vi "SDG60ConfBurst2.vi"(0 "VISA resource name":refnum<visa-resource-name>="USB0::0xF4EC::0x1101::SDG6XEBC5R0119::INSTR", 1 "Trg/Gate Polarity 0: Rise/Pos":u16(ring) items=["Positive", "Negative"], 2 "Triggered/Gated: (0:Triggered)":i32(ring) items=["Triggered", "Gated"], 3 "TRG/Gate Source (0: Internal)":i32(ring) items=["Internal", "External", "Manual"], 5 "Enable Burst (T: Enable)":bool=TRUE, 7 "Channel (1:Channel 1)":i32(ring)=1 items=["Channel 1"=1, "Channel 2"=2], 9 "Start Phase (0.0 degrees)":dbl min=0.0 max=360.0 format="%#.15g", 10 "Burst Period (s)":dbl=1.352e-06, 11 "error in (no error)":errorcluster, 12 "Burst Delay (1.352 us)":dbl=1.352e-06, 13 "Burst Cycle (0: N-Cycle)":u16(ring) items=["N-Cycle", "Infinite"], 14 "Number of Cycles":i32=1) -> (4 "VISA resource name out":refnum<visa-resource-name>, 15 "error out":errorcluster)   [LabVIEW 2018]
panel:
  out "String":string
  # "Note: Ext TRG input is the same as output. TRG/Gate ext input has \nint pull up"
  # "Trigger values can't be changed\nTrigger High: 2-5.5V\nTrigger Low: -0.5-0.8V"
  # "Only positive works as it should\nSetting negative, still responds to rising edge and gives twice\nthe number of burst cycles with a delay. Don't use negative"
  # "Manual not possible in Gate, so\nauto sets to EXT"
  # "Range 1us-110ks. Min depends on freq\nValid and effective only for internal trig setting.\nAffects the period in external trg mode"
  # "Res: 0.1degrees\nRange: -280..+280 deg"
  # "Range: 1.352us-100s\nLimited by frequency\n6 digits precision"
  # "Burst delay also works as a delay with Gate via front panel Delay from triggered mode will be kept in gated mode. To change delay in gated, first need \nto set to triggered with delay time, then switch to gated"
  # "Non-standard behaviour!!: triggers are received while playing out a burst and lead to output of further partial bursts!! Some of these burst appear after burst period setting."
  # "Range: 1-2^31"
  # "When in external finite burst mode there is also a burst counter.\nIf set to >1 will produce multiple bursts with burst period that is\na leftover from triggered mode settnig. Default is 1, not controllable\nwithout using VKeys. Period is also not directly controllable."
  # "When in inf burst mode and ext triggered, the burst will start\nimmediately upon setting up  if external input is HI.\nSwitching output on and off resets inf burst."
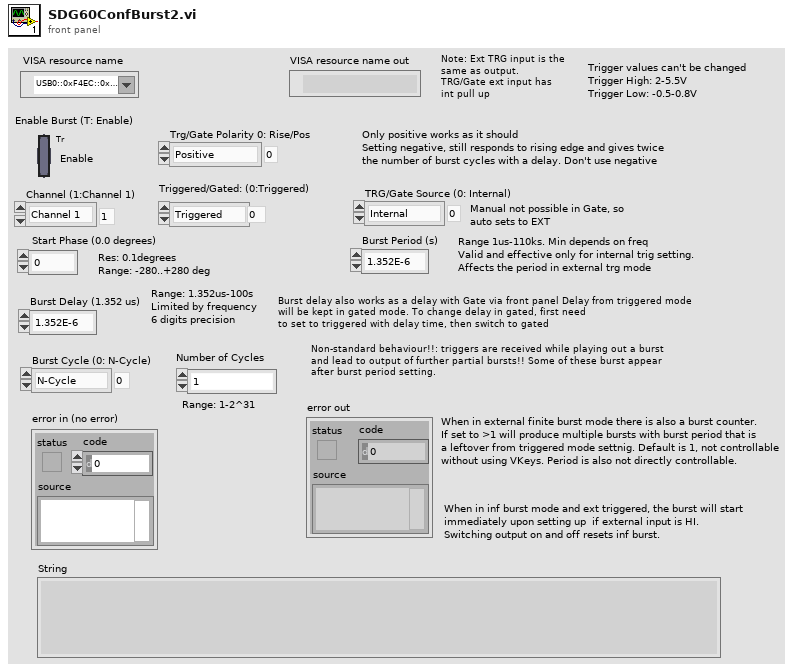
[diagram p1: front panel]
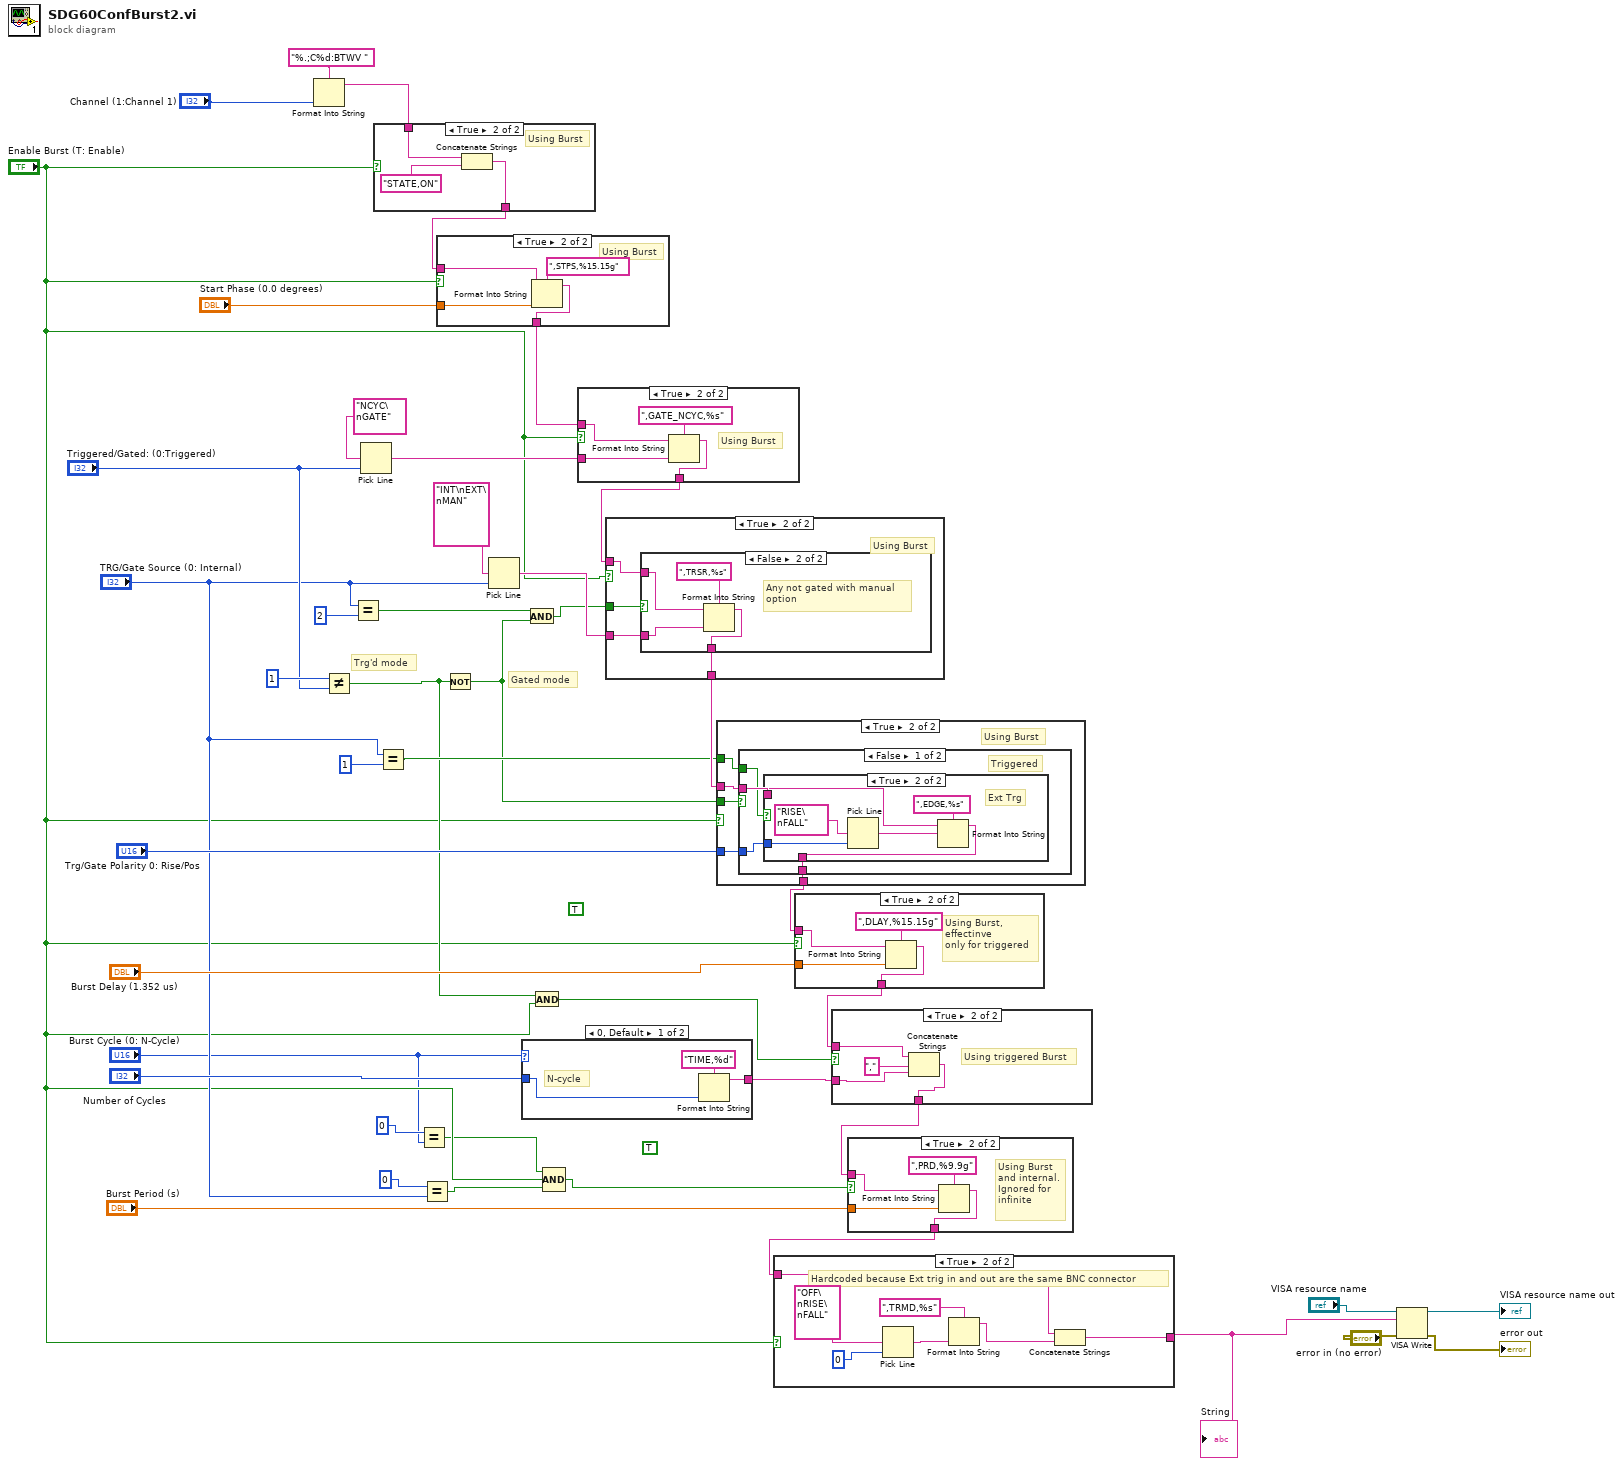
[diagram p0: block diagram]
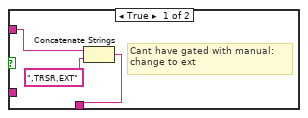
[diagram p4: hidden frame]
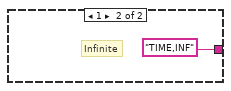
[diagram p6: hidden frame]
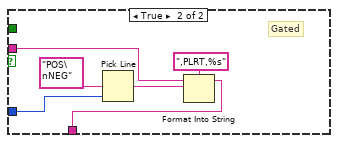
[diagram p10: hidden frame]
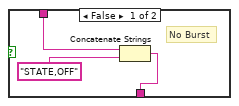
[diagram p14: hidden frame]
diagram:
  (unwired) TRUE
  (unwired) TRUE
  # "Trg'd mode"
  # "Gated mode"
  n1 = Format Into String(format string="%.;C%d:BTWV ", "Channel (1:Channel 1)") -> (resulting string=w42:string)  [unwired: 2 in, 1 out]
  n2 = Not Equal?(x=1, y="Triggered/Gated: (0:Triggered)") -> (x != y?=w7:bool)
  n3 = Equal?(x="TRG/Gate Source (0: Internal)", y=2) -> (x = y?=w15:bool)
  n4 = Pick Line(multi-line string="NCYC\nGATE", line index="Triggered/Gated: (0:Triggered)") -> (output string=w34:string)  [unwired: 1 in]
  n5 = case shown="True" "Enable Burst (T: Enable)" {
    tunnel: w42 -> [w47 w50]
    tunnel: [w45 w48] -> w41
    frame False {
      # "No Burst"
      n6 = Concatenate Strings(w47, "STATE,OFF") -> (w45:string)
    }
    frame True {
      # "Using Burst"
      n7 = Concatenate Strings(w50, "STATE,ON") -> (w48:string)
    }
  }
  n8 = Equal?(x="TRG/Gate Source (0: Internal)", y=1) -> (x = y?=w11:bool)
  n9 = Equal?(x=0, y="Burst Cycle (0: N-Cycle)") -> (x = y?=w2:bool)
  n10 = Equal?(x=0, y="TRG/Gate Source (0: Internal)") -> (x = y?=w5:bool)
  n11 = case shown="True" "Enable Burst (T: Enable)" {
    tunnel: w41 -> [w51 w54]
    tunnel: [w51 w52] -> w30
    tunnel: "Start Phase (0.0 degrees)" -> [_ w55]
    frame False {
      # "No Burst"
    }
    frame True {
      # "Using Burst"
      n12 = Format Into String(format string=",STPS,%15.15g", initial string=w54, w55) -> (resulting string=w52:string)  [unwired: 1 in, 1 out]
    }
  }
  n13 = Not(x=w7) -> (.not. x?=w9:bool)
  n14 = Pick Line(multi-line string="INT\nEXT\nMAN", line index="TRG/Gate Source (0: Internal)") -> (output string=w21:string)  [unwired: 1 in]
  n15 = case shown="0, Default" "Burst Cycle (0: N-Cycle)" {
    tunnel: [w57 "TIME,INF"] -> w26
    tunnel: "Number of Cycles" -> [w56 _]
    frame 0, Default {
      # "N-cycle"
      n16 = Format Into String(format string="TIME,%d", w56) -> (resulting string=w57:string)  [unwired: 2 in, 1 out]
    }
    frame 1 {
      # "Infinite"
    }
  }
  n17 = And(x=w15, y=w9) -> (x .and. y?=w16:bool)
  n18 = And(x=w7, y="Enable Burst (T: Enable)") -> (x .and. y?=w8:bool)
  n19 = Compound Arithmetic op=AND(w2, "Enable Burst (T: Enable)", w5) -> (w6:bool)
  n20 = case shown="True" "Enable Burst (T: Enable)" {
    tunnel: w30 -> [w60 w64]
    tunnel: [w60 w63] -> w18
    tunnel: w34 -> [_ w61]
    frame False {
      # "No Burst"
    }
    frame True {
      # "Using Burst"
      n21 = Format Into String(format string=",GATE_NCYC,%s", initial string=w64, w61) -> (resulting string=w63:string)  [unwired: 1 in, 1 out]
    }
  }
  n22 = case shown="True" "Enable Burst (T: Enable)" {
    tunnel: w18 -> [w65 w68]
    tunnel: [w65 w69] -> w17
    tunnel: w21 -> [_ w67]
    tunnel: w16 -> [_ w66]
    frame False {
      # "No Burst"
    }
    frame True {
      # "Using Burst"
      n23 = case shown="False" w66 {
        tunnel: [w72 w76] -> w69
        tunnel: w68 -> [w71 w74]
        tunnel: w67 -> [_ w73]
        frame True {
          # "Cant have gated with manual: \nchange to ext"
          n24 = Concatenate Strings(w71, ",TRSR,EXT") -> (w72:string)
        }
        frame False {
          # "Any not gated with manual\noption"
          n25 = Format Into String(format string=",TRSR,%s", initial string=w74, w73) -> (resulting string=w76:string)  [unwired: 1 in, 1 out]
        }
      }
    }
  }
  n26 = case shown="True" "Enable Burst (T: Enable)" {
    tunnel: w17 -> [w77 w82]
    tunnel: [w77 w81] -> w29
    tunnel: "Trg/Gate Polarity 0: Rise/Pos" -> [_ w80]
    tunnel: w9 -> [_ w79]
    tunnel: w11 -> [_ w78]
    frame False {
      # "No Burst"
    }
    frame True {
      # "Using Burst"
      n27 = case shown="False" w79 {
        tunnel: w82 -> [w86 w99]
        tunnel: [w84 w98] -> w81
        tunnel: w80 -> [w85 w96]
        tunnel: w78 -> [w83 _]
        frame False {
          # "Triggered"
          n28 = case shown="True" w83 {
            tunnel: w86 -> [w87 w90]
            tunnel: w85 -> [_ w89]
            tunnel: [w87 w88] -> w84
            frame False {
              # "Triggered but not on external"
            }
            frame True {
              # "Ext Trg"
              n29 = Pick Line(multi-line string="RISE\nFALL", line index=w89) -> (output string=w93:string)  [unwired: 1 in]
              n30 = Format Into String(format string=",EDGE,%s", initial string=w90, w93) -> (resulting string=w88:string)  [unwired: 1 in, 1 out]
            }
          }
        }
        frame True {
          # "Gated"
          n31 = Pick Line(multi-line string="POS\nNEG", line index=w96) -> (output string=w95:string)  [unwired: 1 in]
          n32 = Format Into String(format string=",PLRT,%s", initial string=w99, w95) -> (resulting string=w98:string)  [unwired: 1 in, 1 out]
        }
      }
    }
  }
  n33 = case shown="True" "Enable Burst (T: Enable)" {
    tunnel: w29 -> [w100 w104]
    tunnel: "Burst Delay (1.352 us)" -> [_ w102]
    tunnel: [w100 w101] -> w28
    frame False {
      # "No Burst\nand/or gated"
    }
    frame True {
      # "Using Burst,\neffectinve\nonly for triggered"
      n34 = Format Into String(format string=",DLAY,%15.15g", initial string=w104, w102) -> (resulting string=w101:string)  [unwired: 1 in, 1 out]
    }
  }
  n35 = case shown="True" w8 {
    tunnel: w28 -> [w105 w109]
    tunnel: w26 -> [_ w107]
    tunnel: [w105 w106] -> w25
    frame False {
      # "No Burst"
    }
    frame True {
      # "Using triggered Burst"
      n36 = Concatenate Strings(w109, ",", w107) -> (w106:string)
    }
  }
  n37 = case shown="True" w6 {
    tunnel: w25 -> [w110 w114]
    tunnel: "Burst Period (s)" -> [_ w112]
    tunnel: [w110 w111] -> w13
    frame False {
      # "No Burst\nand/or gated"
    }
    frame True {
      # "Using Burst\nand internal.\nIgnored for\ninfinite"
      n38 = Format Into String(format string=",PRD,%9.9g", initial string=w114, w112) -> (resulting string=w111:string)  [unwired: 1 in, 1 out]
    }
  }
  n39 = case shown="True" "Enable Burst (T: Enable)" {
    tunnel: [w115 w117] -> w14
    tunnel: w13 -> [w115 w116]
    frame False {
    }
    frame True {
      # "Hardcoded because Ext trig in and out are the same BNC connector"
      n40 = Pick Line(multi-line string="OFF\nRISE\nFALL", line index=0) -> (output string=w122:string)  [unwired: 1 in]
      n41 = Format Into String(format string=",TRMD,%s", w122) -> (resulting string=w121:string)  [unwired: 2 in, 1 out]
      n42 = Concatenate Strings(w116, w121) -> (w117:string)
    }
  }
  "String" <- w14
  n43 = VISA Write(VISA resource name="VISA resource name", write buffer=w14, error in (no error)="error in (no error)") -> (VISA resource name out=→"VISA resource name out":refnum<visa-resource-name>, error out=→"error out":errorcluster)  [unwired: 1 out]
